vi "niRFSysCalReader Fetch Instrument Temp.vi"(8 "error in":errorcluster, 9 "Level (dBm)":dbl, 10 "Frequency (Hz)":dbl, 11 "niRFSysCalReader Handle":T1) -> (0 "error out":errorcluster, 2 "Temperature (deg C)":dbl, 3 "niRFSysCalReader Handle out":T1)   [LabVIEW 2017, in "niRFSysCalReader.lvlib"]
doc: "Returns the instrument's temperature, when it was calibrated at the specified frequency and power / ref level.\n\n<b>Note:</b> If the Path Type is a TXPath this refers to the signal generator's temperature. If the Path Type is a RXPath this refers to the signal analyzer's temperature."
uses:
  niRFSysCalReader.lvlib
  INCLUDES/niRFSysCalReader Handle.ctl
  INCLUDES/niRFSysCalReader Core States.ctl
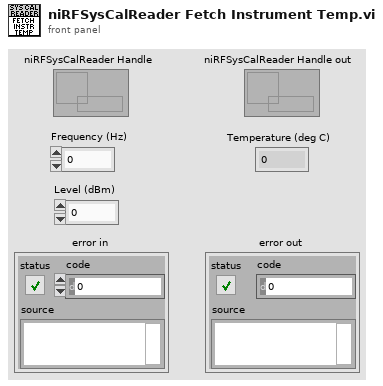
[diagram p1: front panel]
types:
  T1 = typedef "niRFSysCalReader.lvlib/niRFSysCalReader Handle.ctl" = refnum<data-value>
  T2 = typedef "niRFSysCalReader.lvlib/niRFSysCalReader Core States.ctl" = enum16{"Initialize", "Interpolator State", "Add CalData", "Get CalData", "Remove Pathloss", "Close"}
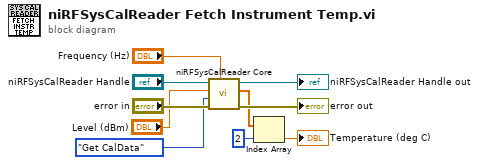
[diagram p0: block diagram]
diagram:
  n1 = call "niRFSysCalReader Core.vi"("Frequency (Hz)"="Frequency (Hz)", "error in"="error in", "niRFSysCalReader State"=niRFSysCalReader_Core_States."Get CalData" ("Cal Storage"), "Power (dBm)"="Level (dBm)", "niRFSysCalReader Handle"="niRFSysCalReader Handle") -> ("error out"=→"error out":errorcluster, "CalData Out"=w2:dbl[], "niRFSysCalReader Handle out"=→"niRFSysCalReader Handle out":T1)  [unwired: 4 in]
  n2 = Index Array(array=w2, index=2) -> (element=→"Temperature (deg C)":dbl)
